vi "LLB Pre-Build CHM Build.vi"(6 "Top Level/Always Included VIs":path[](array[path]), 7 "Main Destination Path":path, 9 "Target Name":string, 10 "Build Specification Name":string, 11 "Project Path":path) -> (0 "error out":errorcluster)   [LabVIEW 2019]
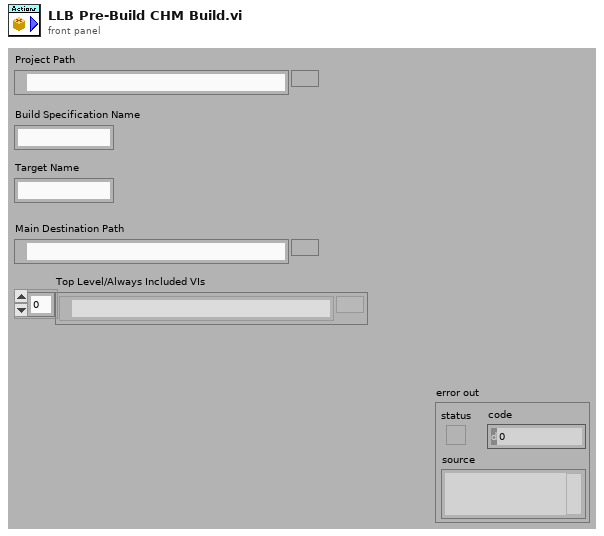
[diagram p1: front panel]
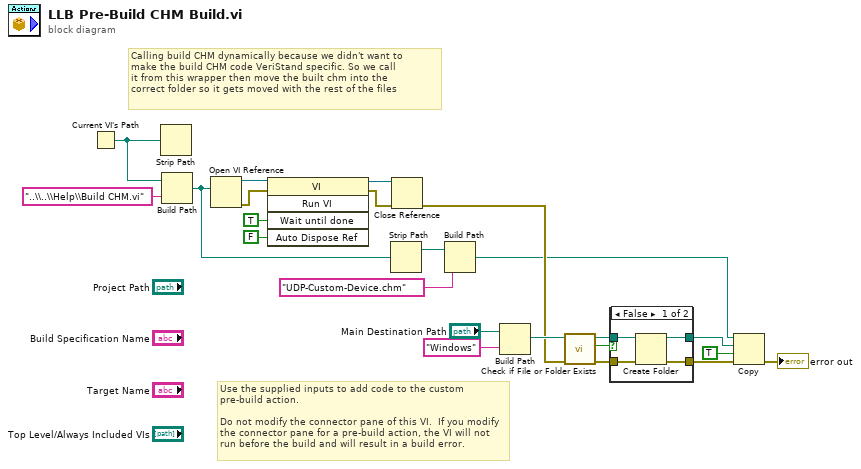
[diagram p0: block diagram]
diagram:
  # "Calling build CHM dynamically because we didn't want to \nmake the build CHM code VeriStand specific. So we call\nit from this wrapper then move the built chm into the\ncorrect folder so it gets moved with the rest of the files"
  # "Use the supplied inputs to add code to the custom pre-build action.\n\nDo not modify the connector pane of this VI.  If you modify the connector pane for a pre-build action, the VI will not run before the build and will result in a build error."
  n1 = Current VI's Path() -> (path=w2:path)
  n2 = Strip Path(path=w2) -> ()  [unwired: 2 out]
  n3 = Build Path(base path=w2, name or relative path="..\\..\\Help\\Build CHM.vi") -> (appended path=w16:path)
  n4 = Open VI Reference(vi path=w16) -> (vi reference=w22:refnum<vi>, error out=w21:errorcluster)  [unwired: 5 in]
  n5 = invoke class="VI" method="Run VI"(reference=w22, error in=w21, "Wait until done"=TRUE ("Wait Until Done"), "Auto Dispose Ref"=FALSE ("Auto Dispose Reference")) -> (reference out=w18:refnum<vi>, error out=w17:errorcluster)  [unwired: 1 in, 3 out]
  n6 = Strip Path(path=w16) -> (stripped path=w15:path)  [unwired: 1 out]
  n7 = Close Reference(reference=w18, error in (no error)=w17) -> (error out=w11:errorcluster)
  n8 = Build Path(base path=w15, name or relative path="UDP-Custom-Device.chm" ("string")) -> (appended path=w4:path)
  n9 = Build Path(base path="Main Destination Path", name or relative path="Windows") -> (appended path=w12:path)
  n10 = call <vilib>:"Check if File or Folder Exists.vi"("error in (no error)"=w11, "path"=w12) -> ("error out"=w8:errorcluster, "file or folder exists?"=w10:bool, "dup path"=w9:path)  [unwired: 7 in]
  n11 = case shown="False" w10 {
    tunnel: w9 -> [w26 w29]
    tunnel: w8 -> [w27 w28]
    tunnel: [w25 w29] -> w6
    tunnel: [w24 w28] -> w7
    frame False {
      n12 = Create Folder(path (use dialog)=w26, error in=w27) -> (created path=w25:path, error out=w24:errorcluster)  [unwired: 1 in, 1 out]
    }
    frame True {
    }
  }
  n13 = Copy(8:w7, 9:TRUE ("overwrite (F)"), 10:w6, 11:w4) -> (0:→"error out":errorcluster)  [unwired: 1 in, 2 out]
